vi "Image.vi"(10 "data":dbl[][](array[numeric]), 11 "Draw Area Size":T1) -> (0 "Rectangle.bottom":i16, 1 "Rectangle.right":i16, 2 "new picture":picture, 3 "ZoomFactor":dbl)   [LabVIEW 2021]
uses:
  <vilib>/Utility/miscctls.llb/LVBoundsTypeDef.ctl
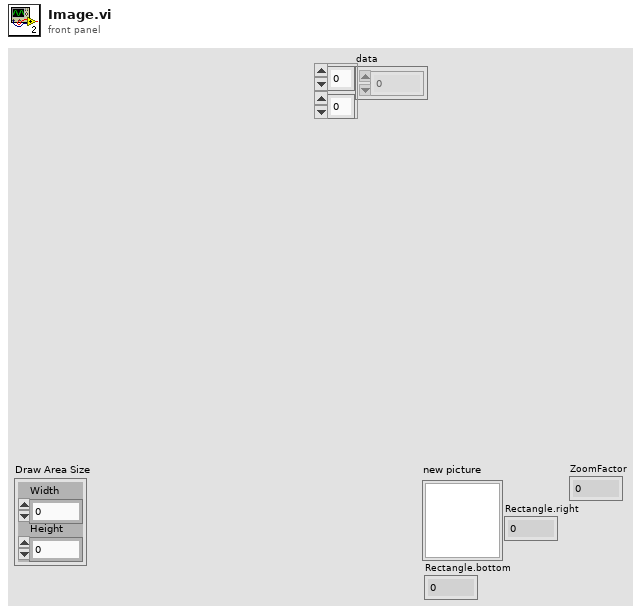
[diagram p1: front panel]
types:
  T1 = typedef "LVBoundsTypeDef.ctl" = cluster{"Width":u32, "Height":u32}
  T2 = typedef "imagedata.ctl" = cluster{"image type":i32, "image depth":i32, "image":u8[], "mask":u8[], "colors":u32[], "Rectangle":cluster{"left":i16, "top":i16, "right":i16, "bottom":i16}}
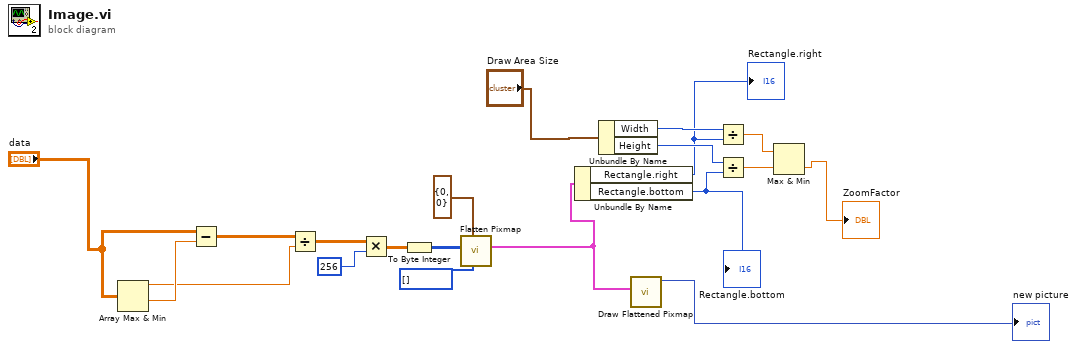
[diagram p0: block diagram]
diagram:
  n1 = Array Max & Min(array="data") -> (max value=w18:dbl, min value=w20:dbl)  [unwired: 2 out]
  n2 = Subtract(x="data", y=w20) -> (x-y=w19:dbl[][])
  n3 = Divide(x=w19, y=w18) -> (x/y=w17:dbl[][])
  n4 = Multiply(x=w17, y=256) -> (x*y=w15:dbl[][])
  n5 = To Byte Integer(number=w15) -> (8bit integer=w14:i8[][])
  n6 = call <vilib>:"Flatten Pixmap.vi"("colors"=u32[] [], "top left"=cluster{"x":i16, "y":i16} {"x"=0, "y"=0}, "8-bit pixmap"=w14) -> ("image data"=w4:T2)  [unwired: 8 in]
  n7 = Unbundle By Name(w4) -> ("Rectangle.right"=w6:i16, "Rectangle.bottom"=w5:i16)
  "Rectangle.bottom" <- w5
  "Rectangle.right" <- w6
  n8 = Unbundle By Name("Draw Area Size") -> ("Width"=w10:u32, "Height"=w9:u32)
  n9 = call <vilib>:"Draw Flattened Pixmap.vi"("image data"=w4) -> ("new picture"=→"new picture":picture)  [unwired: 8 in]
  n10 = Divide(x=w10, y=w6) -> (x/y=w8:dbl)
  n11 = Divide(x=w9, y=w5) -> (x/y=w7:dbl)
  n12 = Max & Min(x=w8, y=w7) -> (min(x,y)=→"ZoomFactor":dbl)  [unwired: 1 out]
